vi "0025ConfusingSwitchesAns.vi"() -> ()   [LabVIEW 2010]
panel:
  out "The Light":bool
  in  "C":bool
  in  "B":bool
  in  "A":bool
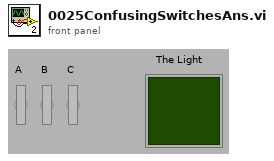
[diagram p1: front panel]
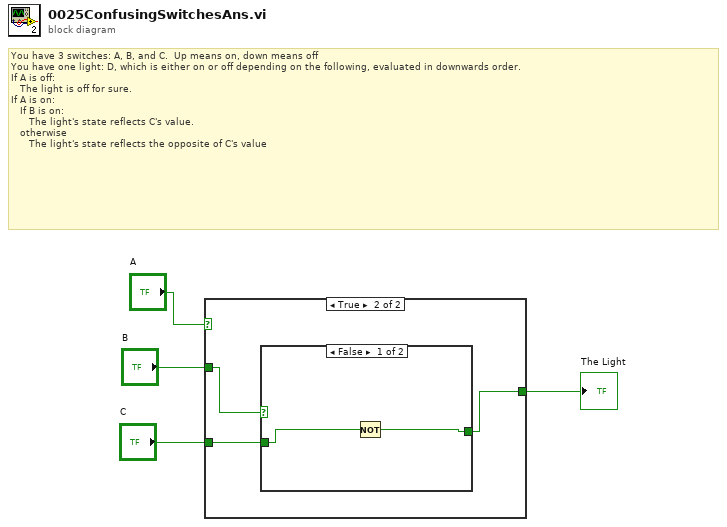
[diagram p0: block diagram]
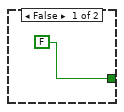
[diagram p2: hidden frame]
diagram:
  # "You have 3 switches: A, B, and C.  Up means on, down means off\nYou have one light: D, which is either on or off depending on the following, evaluated in downwards order.\nIf A is off: \n   The light is off for sure.\nIf A is on:\n   If B is on:\n      The light's state reflects C's value.\n   otherwise\n      The light's state reflects the opposite of C's value"
  n1 = case shown="True" "A" {
    tunnel: "B" -> [_ w8]
    tunnel: "C" -> [_ w7]
    tunnel: [FALSE w6] -> w1
    frame False {
    }
    frame True {
      n2 = case shown="False" w8 {
        tunnel: w7 -> [w10 w11]
        tunnel: [w9 w11] -> w6
        frame False {
          n3 = Not(x=w10) -> (.not. x?=w9:bool)
        }
        frame True {
        }
      }
    }
  }
  "The Light" <- w1
